vi "PKG_IMC_MulLine_Dist.vi"(0 "handle":u32, 1 "tgvel":dbl, 2 "wait":i32, 5 "dist":i32, 7 "axisNum":i32, 9 "segNum":i32, 12 "endvel":dbl, 13 "fifo":i32) -> (4 "handle out":u32, 6 "dist out":i32, 8 "function return":i32)   [LabVIEW 2011, in "IMC_Pkg4xxx.lvlib"]
doc: "PKG_IMC_MulLine_Dist (IMC_HANDLE handle, long* dist, int axisNum, int segNum, double tgvel, double endvel, int wait, int fifo);"
uses:
  IMC_Pkg4xxx.lvlib
  IMC_Pkg4xxx.dll
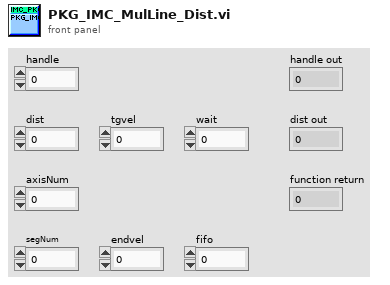
[diagram p1: front panel]
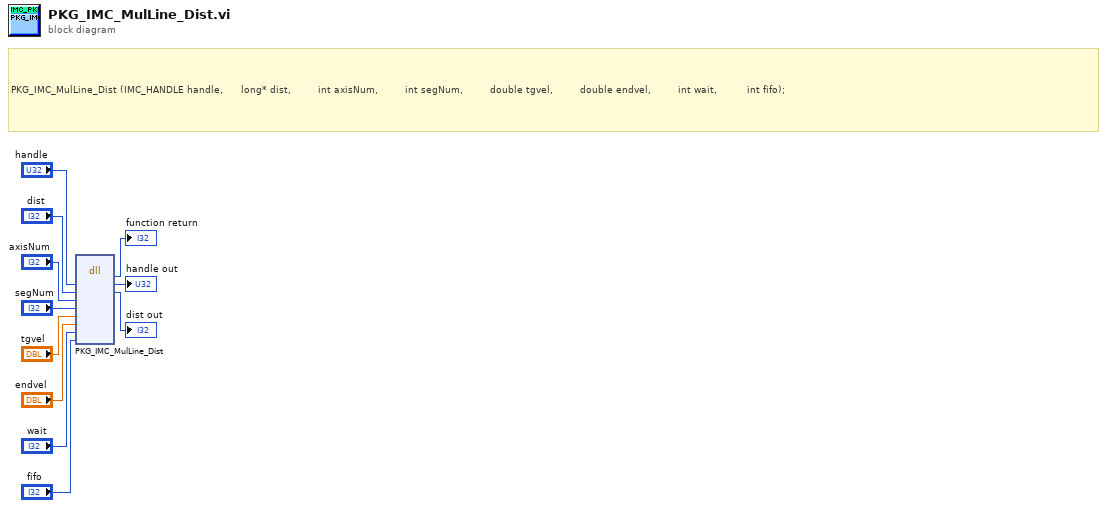
[diagram p0: block diagram]
diagram:
  # "PKG_IMC_MulLine_Dist (IMC_HANDLE handle, \t\t\t\t\tlong* dist, \t\t\t\t\t\t\t\tint axisNum, \t\t\t\t\t\t\t\tint segNum, \t\t\t\t\t\t\t\tdouble tgvel, \t\t\t\t\t\t\t\tdouble endvel, \t\t\t\t\t\t\t\tint wait, \t\t\t\t\t\t\t\t\tint fifo);"
  n1 = dll-call lib="PTH1mabs F光盘刻录\niMC MotionIMCNet_V4.0IMCAppincLabviewIMC_PKG4xxxIMC_PKG4xxx\nIMC_Pkg4xxx.*" fn="PKG_IMC_MulLine_Dist"("handle"="handle", "dist"="dist", "axisNum"="axisNum", "segNum"="segNum", "tgvel"="tgvel", "endvel"="endvel", "wait"="wait", "fifo"="fifo") -> (→"function return":i32, "handle"=→"handle out":u32, "dist"=→"dist out":i32)  [unwired: 9 in, 2 out]
